vi "ReadInputMap.vi"(8 "Error In":errorcluster, 11 "object in":refnum<class "Conjunction.lvclass">) -> (0 "Error Out":errorcluster, 2 "Input Map":map{string, bool}(c390), 3 "object out":refnum<class "Conjunction.lvclass">)   [LabVIEW 2021, in "Conjunction.lvclass"]
uses:
  Conjunction.lvclass
  Conjunction.lvclass/Conjunction.ctl
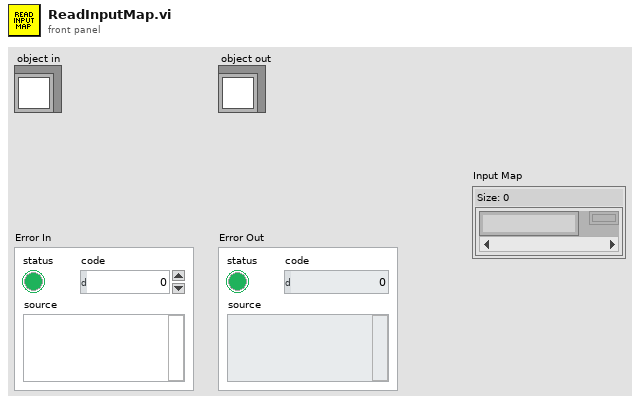
[diagram p1: front panel]
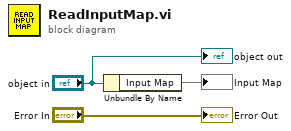
[diagram p0: block diagram]
diagram:
  n1 = Unbundle By Name("object in") -> ("Input Map"=→"Input Map":map{string, bool})
  "Error Out" <- "Error In"
  "object out" <- "object in"
